vi "Get position 2.vi"(6 "Motor params":T1={"Tipo"=2, "Dirección"=1, "N°. Pasos"=1, "Frecuencia (Hz)"=100, "Tipo de paso"=100} {"Tipo de paso" items=["", "Medio paso", "Paso completo"]; "Dirección" items=["", "Izquierda", "Derecha"]; "Tipo" items=["", "Unipolar", "Bipolar"]}, 7 "mm/step":dbl=0.0025, 8 "error in (no error)":errorcluster, 10 "Position in":dbl, 11 "VISA resource name in":refnum<visa-resource-name>) -> (0 "error out":errorcluster, 1 "End?":bool, 2 "Positions out":dbl, 3 "VISA Refnum out":refnum<visa-resource-name>)   [LabVIEW 2020, in "Control de MaP.lvlib"]
doc: "Asks the MCU for the current position of the motor. The position is returned as a string and interpreted in steps, set mm/step to convert to proper units. Once the current position is returned, the MCU resets the internal value to zero.\n\nNote: the MCU does not keep track of the absolute position, it befalls on the developer to store and manage the corresponding variable inside LabVIEW. For such purpose, the nodes Position in and Position out are provided."
uses:
  Control de MaP.lvlib
  Controls/Command to motor.ctl
  <vilib>/Instr/_visa.llb/VISA Flush IO Buffer Mask.ctl
  Write--command.vi
panel:
  out "Command out":string
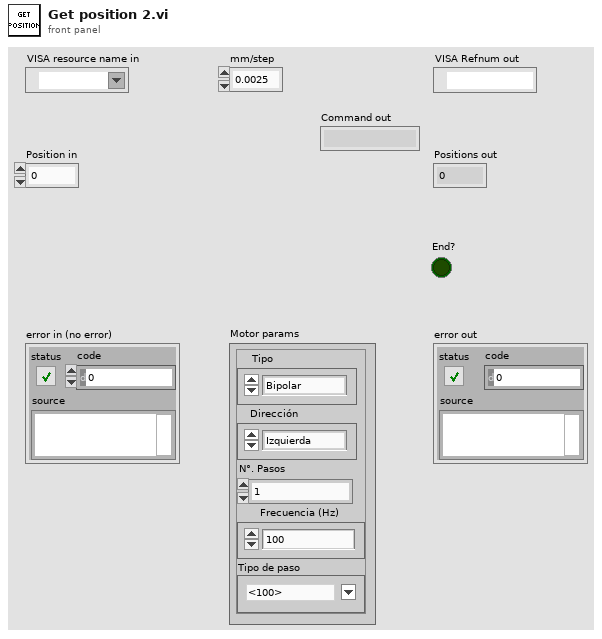
[diagram p1: front panel]
types:
  T1 = typedef "Control de MaP.lvlib/Command to motor.ctl" = cluster{"Tipo":u8, "Dirección":u8, "N°. Pasos":u16, "Frecuencia (Hz)":u8, "Tipo de paso":u8}
  T2 = typedef "VISA Flush IO Buffer Mask.ctl" = u16
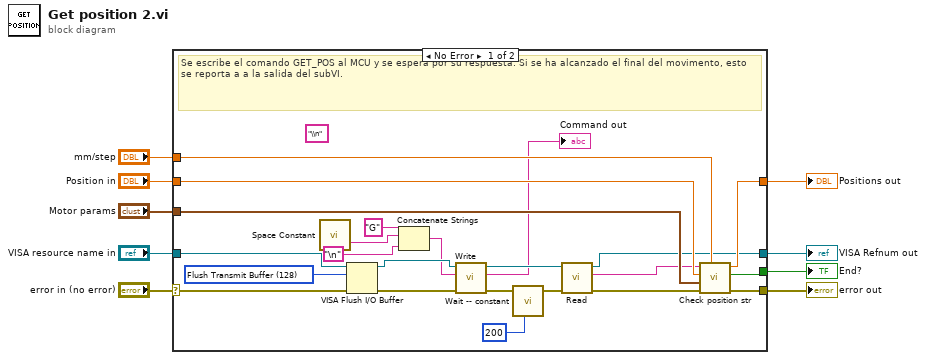
[diagram p0: block diagram]
diagram:
  n1 = case shown="No Error" "error in (no error)" {
    selector: "error in (no error)" -> [w20 w33]
    tunnel: [w32 w35] -> w9
    tunnel: "Position in" -> [w31 w35]
    tunnel: [w23 w33] -> w8
    tunnel: "Motor params" -> [w30 _]
    tunnel: "mm/step" -> [w29 _]
    tunnel: "VISA resource name in" -> [w18 w34]
    tunnel: [w24 w34] -> w2
    tunnel: [w21 _] -> w1
    frame No Error {
      (unwired) "\\n" ("string")
      w16 = T2 128 items=["Flush Receive Buffer"=16, "Write Transmit Buffer to Device"=32, "Flush Receive Buffer (No I/O)"=64, "Flush Transmit Buffer"=128] ("Mask")
      # "Se escribe el comando GET_POS al MCU y se espera por su respuesta. Si se ha alcanzado el final del movimento, esto se reporta a a la salida del subVI."
      n2 = call <vilib>:"Space Constant.vi"() -> ("String"=w10:string)
      n3 = VISA Flush I/O Buffer(VISA resource name=w18, mask (16)=w16, error in (no error)=w20) -> (VISA resource name out=w17:refnum<visa-resource-name>, error out=w19:errorcluster)
      n4 = Concatenate Strings("G" ("Command"), w10, "\n") -> (w13:string)
      n5 = call-poly "Write.vi"("error in (no error)"=w19, "Command"=w13, "VISA resource name"=w17) -> ("error out"=w27:errorcluster, "Command out"=→"Command out":string, "VISA resource name out"=w28:refnum<visa-resource-name>)  [unwired: 6 in]
      n6 = call "Wait -- constant.vi"("error in (no error)"=w27, "wait (100 ms)"=u32 200) -> ("error out"=w26:errorcluster)  [unwired: 5 in]
      n7 = call "Read.vi"("error in (no error)"=w26, "VISA resource name"=w28) -> ("error out"=w22:errorcluster, "Recibo de Datos"=w25:string, "VISA resource name out"=w24:refnum<visa-resource-name>)  [unwired: 6 in, 1 out]
      n8 = call "Check position str.vi"("mm/step"=w29, "error in (no error)"=w22, "Motor params"=w30, "Position in"=w31, "String read"=w25) -> ("error out"=w23:errorcluster, "End?"=w21:bool, "Position out"=w32:dbl)  [unwired: 4 in]
    }
    frame Error {
    }
  }
  "Positions out" <- w9
  "error out" <- w8
  "VISA Refnum out" <- w2
  "End?" <- w1
